vi "噪声子VI输入波形.vi"(2 "输入波形":waveform(dbl) caption="波形", 3 "噪声选择":enum16{"无", "均匀白噪声", "高斯噪声", "周期性随机噪声"}(ring), 4 "幅值":dbl) -> (1 "波形图":waveform(dbl)(graph))   [LabVIEW 2017]
uses:
  <vilib>/measure/NI_MABase.lvlib
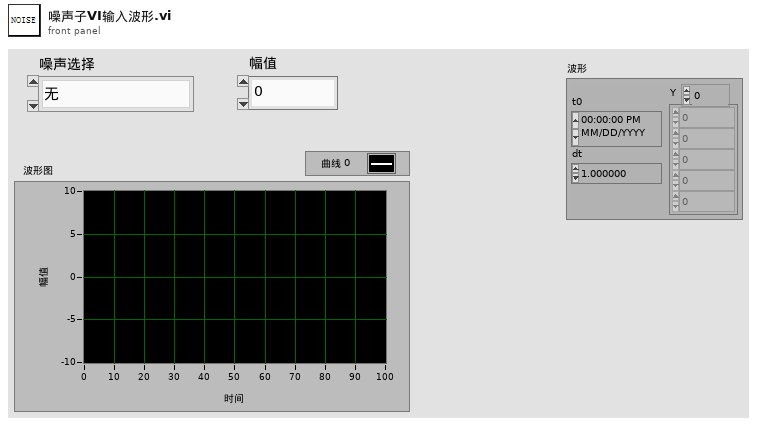
[diagram p1: front panel]
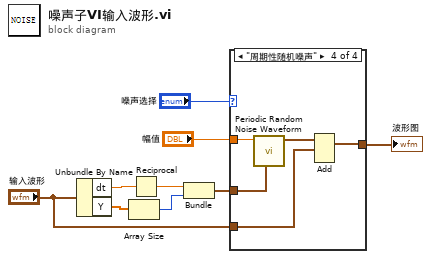
[diagram p0: block diagram]
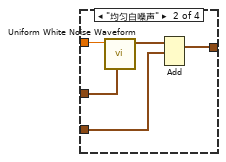
[diagram p3: hidden frame]
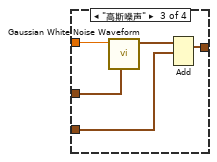
[diagram p4: hidden frame]
diagram:
  n1 = Unbundle By Name("输入波形") -> ("dt"=w6:dbl, "Y"=w5:dbl[])
  n2 = Array Size(array=w5) -> (size(s)=w3:i32)
  n3 = Reciprocal(x=w6) -> (1/x=w4:dbl)
  n4 = Bundle(w4, w3) -> (w2:cluster{dbl, i32})  [unwired: 1 in]
  n5 = case shown="\"周期性随机噪声\"" "噪声选择" {
    tunnel: "幅值" -> [_ w15 w20 w25]
    tunnel: "输入波形" -> [w10 w12 w17 w22]
    tunnel: [w10 w11 w16 w21] -> w1
    tunnel: w2 -> [_ w14 w19 w24]
    frame "无", Default {
    }
    frame "均匀白噪声" {
      n6 = call <vilib>:"Uniform White Noise Waveform.vi"("sampling info"=w14, "amplitude"=w15) -> ("signal out"=w13:waveform(dbl))  [unwired: 8 in, 1 out]
      n7 = Add(1:w12, 2:w13) -> (0:w11:waveform(dbl))  [unwired: 1 in, 1 out]
    }
    frame "高斯噪声" {
      n8 = call <vilib>:"Gaussian White Noise Waveform.vi"("sampling info"=w19, "standard deviation"=w20) -> ("signal out"=w18:waveform(dbl))  [unwired: 8 in, 1 out]
      n9 = Add(1:w17, 2:w18) -> (0:w16:waveform(dbl))  [unwired: 1 in, 1 out]
    }
    frame "周期性随机噪声" {
      n10 = call <vilib>:"Periodic Random Noise Waveform.vi"("sampling info"=w24, "spectral amplitude"=w25) -> ("signal out"=w23:waveform(dbl))  [unwired: 8 in, 1 out]
      n11 = Add(1:w22, 2:w23) -> (0:w21:waveform(dbl))  [unwired: 1 in, 1 out]
    }
  }
  "波形图" <- w1
